vi "JSON Get.vi"(7 "Default":variant, 8 "error in (no error)":errorcluster, 10 "Root Path ([]=Root)":string[](array[string]), 11 "JSON in":string) -> (0 "error out":errorcluster, 2 "Exists?":bool, 3 "Value":variant)   [LabVIEW 2019, in "labview_json.lvlib"]
doc: "Get an element from the <b>JSON in</b> string. \nIf the element is not found, <b>Default</b> is returned. \nSpecify the <b>Root Path</b> to the nested object key or array index. \nIf <b>Default</b> is not specified, this returns the native JSON types. \n<b>Exists?</b> only returns True if all elements are found.\nCreated by: Ryan Pacini"
uses:
  labview_json.lvlib
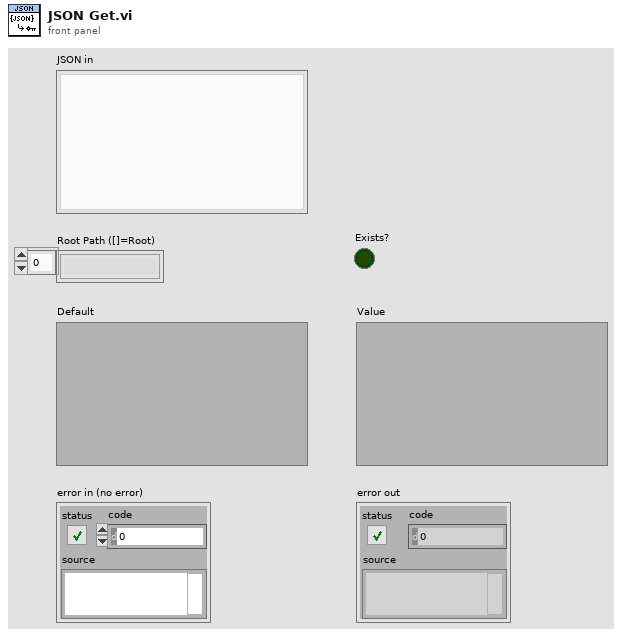
[diagram p1: front panel]
types:
  T1 = typedef "labview_json.lvlib/Element.ctl" = cluster{"Key":string, "Type":T2, "Value":variant, "IsRootPath":bool}
  T2 = typedef "labview_json.lvlib/Element Type.ctl" = enum8{"NULL", "OBJECT", "ARRAY", "BOOL", "INT", "UINT", "FLOAT", "STRING"}
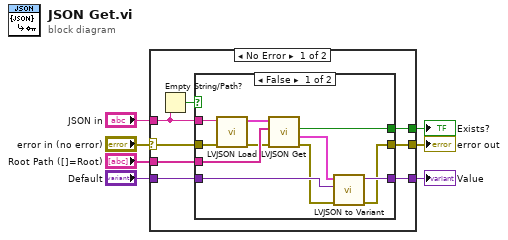
[diagram p0: block diagram]
diagram:
  n1 = case shown="No Error" "error in (no error)" {
    selector: "error in (no error)" -> [w15 w30]
    tunnel: [w10 w30] -> w6
    tunnel: "JSON in" -> [w9 _]
    tunnel: "Root Path ([]=Root)" -> [w14 _]
    tunnel: "Default" -> [w13 w29]
    tunnel: [w12 w29] -> w3
    tunnel: [w11 _] -> w2
    frame No Error {
      n2 = Empty String/Path?(string/path=w9) -> (empty?=w8:bool)
      n3 = case shown="False" w8 {
        tunnel: w15 -> [w26 w28]
        tunnel: w9 -> [w25 _]
        tunnel: w14 -> [w23 _]
        tunnel: w13 -> [w21 w27]
        tunnel: [w20 w27] -> w12
        tunnel: [w18 _] -> w11
        tunnel: [w17 w28] -> w10
        frame False {
          n4 = call "LVJSON Load.vi"("error in (no error)"=w26, "JSON in"=w25) -> ("error out"=w16:errorcluster, "Root Element out"=w24:T1)  [unwired: 8 in]
          n5 = call "LVJSON Get.vi"("error in (no error)"=w16, "Root Path"=w23, "Root Element in"=w24) -> ("error out"=w19:errorcluster, "Element out"=w22:T1, "Exists?"=w18:bool)  [unwired: 5 in, 1 out]
          n6 = call "LVJSON to Variant.vi"("error in (no error)"=w19, "Variant Type"=w21, "Root Element in"=w22) -> ("error out"=w17:errorcluster, "Variant out"=w20:variant)  [unwired: 6 in, 1 out]
        }
        frame True {
        }
      }
    }
    frame Error {
    }
  }
  "error out" <- w6
  "Value" <- w3
  "Exists?" <- w2
